vi "VeriStand DSF.Plugin.Configuration.Get Section Reference.vi"(11 "VeriStand DSF.Plugin.Configuration in":refnum<class "VeriStand DSF.Plugin.Configuration.lvclass">=refnum) -> (2 "Section Ref":T1=18446744073709551615 format="%.0x", 3 "VeriStand DSF.Plugin.Configuration out":refnum<class "VeriStand DSF.Plugin.Configuration.lvclass">)   [LabVIEW 2017, in "Data Sharing Custom Device Engine.lvlib" / "VeriStand DSF.Plugin.Configuration.lvclass"]
uses:
  VeriStand DSF.Plugin.Configuration.lvclass
  <vilib>/NI Veristand/Custom Device API/Custom Device Item Ref.ctl
  VeriStand DSF.Plugin.Configuration.lvclass/VeriStand DSF.Plugin.Configuration.ctl
  <vilib>/NI Veristand/Custom Device API/Custom Device API.lvlib
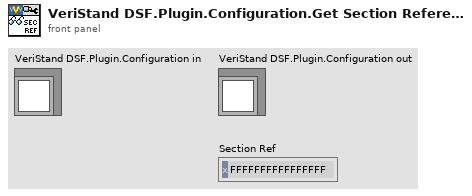
[diagram p1: front panel]
types:
  T1 = typedef "Custom Device API.lvlib/Custom Device Item Ref.ctl" = u64
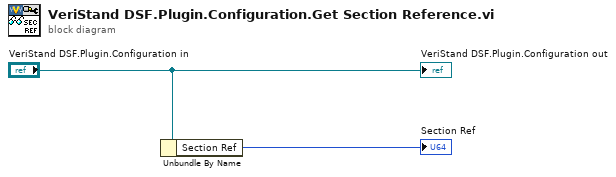
[diagram p0: block diagram]
diagram:
  n1 = Unbundle By Name("VeriStand DSF.Plugin.Configuration in") -> ("Section Ref"=→"Section Ref":T1)
  "VeriStand DSF.Plugin.Configuration out" <- "VeriStand DSF.Plugin.Configuration in"
